vi "ToString.vi"(8 "error in (no error)":errorcluster, 11 "Collection Contains in":refnum<class "Collection Contains.lvclass">) -> (0 "error out":errorcluster, 2 "String":string, 3 "Collection Contains out":refnum<class "Collection Contains.lvclass">)   [LabVIEW 2017, in "Transparent Assertions.lvlib" / "Collection Contains.lvclass"]
doc: "Returns a string representation of the object."
uses:
  Collection Contains.lvclass
  Collection Contains.lvclass/Collection Contains.ctl
  To JSON.vi/c34f3794-71bb-4fc1-98c1-2c7c55f09150.vi
  <vilib>/PNR/JSONtext Object Serialization/Generic Object Serializer/Generic Object Serializer.lvclass
  C:/Program Files/National Instruments/LabVIEW 2017/vi.lib/JDP Science/JSONtext/LVClass Serializer/JSONtext LVClass Serializer.lvclass
  <vilib>/JDP Science/JSONtext/Variant to JSON Text.vi
  Transparent Assertions.lvlib
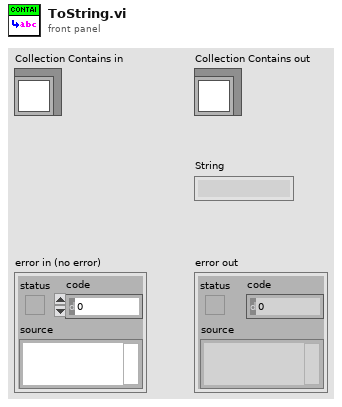
[diagram p1: front panel]
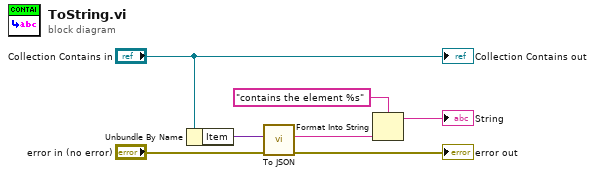
[diagram p0: block diagram]
diagram:
  n1 = Unbundle By Name("Collection Contains in") -> ("Item"=w3:variant)
  n2 = call "To JSON.vi"("error in (no error)"="error in (no error)", "Anything"=w3) -> ("error out"=→"error out":errorcluster, "JSON"=w2:string)  [unwired: 8 in]
  n3 = Format Into String(format string="contains the element %s", w2) -> (resulting string=→"String":string)  [unwired: 2 in, 1 out]
  "Collection Contains out" <- "Collection Contains in"
